vi "Putty send Comand.vi"(0 "Command(s) to Execute":string="ssh almaproc@10.192.1.123 'python /users/almaproc/scripts/testCanMonitor -a test-abm -c 1'") -> ()   [LabVIEW 2010]
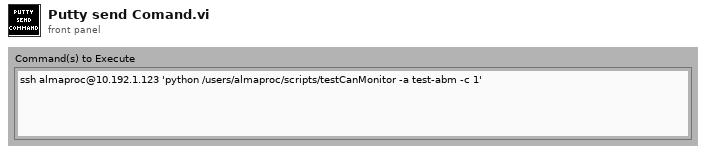
[diagram p1: front panel]
types:
  T1 = enum32{"invalid app kind", "Development System", "Run Time System", "Student Edition", "Embedded LabVIEW", "Evaluation", "Custom"}
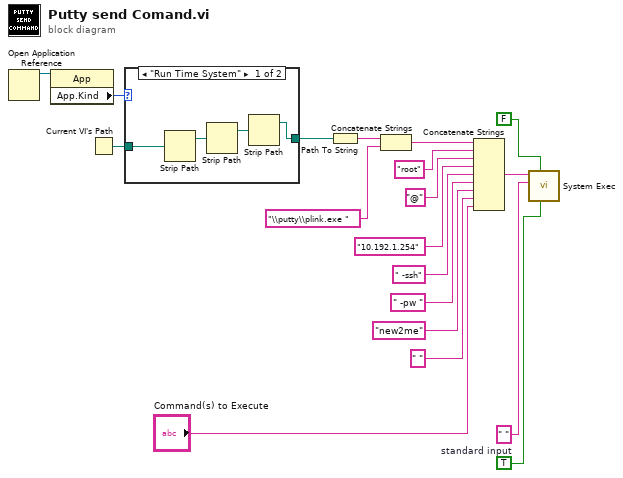
[diagram p0: block diagram]
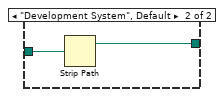
[diagram p2: hidden frame]
diagram:
  w1 = " "  # standard input
  n1 = Open Application Reference() -> (3:w9:refnum<vi>)  [unwired: 4 in, 1 out]
  n2 = property class="App"(reference=w9) -> ("App.Kind"=w10:T1)  [unwired: 1 in, 2 out]
  n3 = Current VI's Path() -> (path=w11:path)
  n4 = case shown="\"Run Time System\"" w10 {
    tunnel: w11 -> [w20 w25]
    tunnel: [w21 w24] -> w12
    frame "Run Time System" {
      n5 = Strip Path(path=w20) -> (stripped path=w22:path)  [unwired: 1 out]
      n6 = Strip Path(path=w22) -> (stripped path=w23:path)  [unwired: 1 out]
      n7 = Strip Path(path=w23) -> (stripped path=w21:path)  [unwired: 1 out]
    }
    frame "Development System", Default {
      n8 = Strip Path(path=w25) -> (stripped path=w24:path)  [unwired: 1 out]
    }
  }
  n9 = Path To String(path=w12) -> (string=w15:string)
  n10 = Concatenate Strings(w15, "\\putty\\plink.exe " ("command line")) -> (w14:string)
  n11 = Concatenate Strings(w14, "root" ("Username"), "@" ("string"), "10.192.1.254" ("Host"), " -ssh", " -pw " ("string"), "new2me" ("Password"), " " ("string"), "Command(s) to Execute") -> (w8:string)
  n12 = call <vilib>:"System Exec.vi"("run minimized? (F)"=TRUE ("Hide DOS\nWindow?"), "wait until completion? (T)"=FALSE, "standard input"=w1, "command line"=w8) -> ()  [unwired: 2 in, 6 out]
